vi "Limit Switch.vi"(10 "Input":dbl) -> (2 "Output":dbl)   [LabVIEW 2013]
uses:
  Robot Global Data.vi
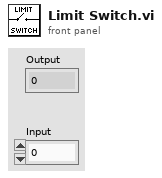
[diagram p1: front panel]
types:
  T1 = typedef "Robot Info Typedef.ctl" = cluster{"Arm Info":T2, "Shooter Info":T3}
  T2 = typedef "Arm Info Typedef.ctl" = cluster{"Current Arm Position":dbl, "Arm Bottom Limit Switch":bool, "Arm Top Limit Switch":bool}
  T3 = typedef "Shooter Info Typedef.ctl" = cluster{"Shooter At Full":bool}
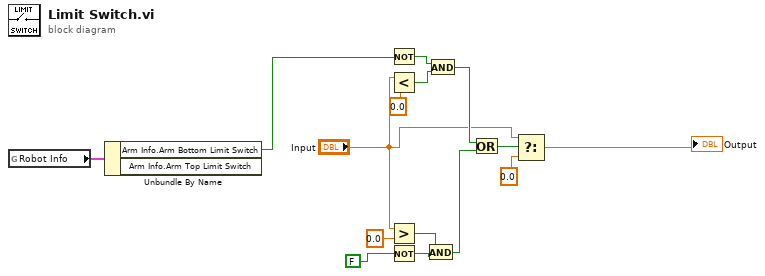
[diagram p0: block diagram]
diagram:
  n1 = global read "Robot Global Data.vi" "Robot Info"() -> (w4:T1)
  n2 = Unbundle By Name(w4) -> ("Arm Info.Arm Bottom Limit Switch"=w3:bool)  [unwired: 1 out]
  n3 = Not(x=w3) -> (.not. x?=w11:bool)
  n4 = Less?(x="Input", y=0.0) -> (x < y?=w12:bool)
  n5 = Greater?(x="Input", y=0.0) -> (0:w14:bool)
  n6 = Not(x=FALSE) -> (.not. x?=w15:bool)
  n7 = And(x=w14, y=w15) -> (x .and. y?=w2:bool)
  n8 = And(x=w11, y=w12) -> (x .and. y?=w10:bool)
  n9 = Or(x=w10, y=w2) -> (x .or. y?=w9:bool)
  n10 = Select(t="Input", s=w9, f=0.0 ("y")) -> (s? t:f=→"Output":dbl)
